vi "DLLPath.vi"(11 "DLL Path In":path) -> (3 "DLL Path Out":path)   [LabVIEW 2024, in "SDL3.lvlib"]
uses:
  SDL3.lvlib
panel:
  in  "Mode (Get)":enum16{"Get", "Set"}(ring)
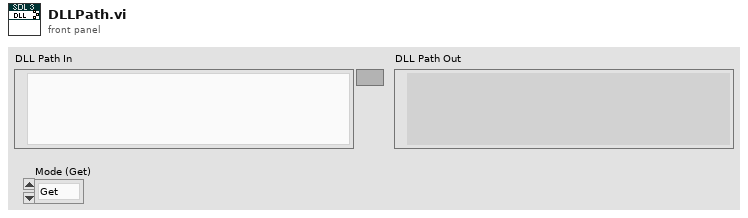
[diagram p1: front panel]
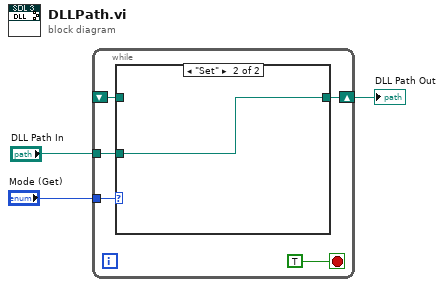
[diagram p0: block diagram]
diagram:
  n1 = while {
    tunnel: "Mode (Get)" -> [w7]
    shift-right: [w6] -> w1
    shift-left: _ -> [w4]
    tunnel: "DLL Path In" -> [w5]
    stop <- TRUE stop-if-true
    n2 = case shown="\"Set\"" w7 {
      tunnel: [w9 w10] -> w6
      tunnel: w5 -> [_ w10]
      tunnel: w4 -> [w9 _]
      frame "Get", Default {
      }
      frame "Set" {
      }
    }
  }
  "DLL Path Out" <- w1
